vi "Empty.vi"(0 "object in":refnum<class "CetoniPump.lvclass">, 2 "index":i32, 5 "error in (no error)":errorcluster) -> (14 "object out":refnum<class "CetoniPump.lvclass">, 19 "error out":errorcluster)   [LabVIEW 2023, in "CetoniPump.lvclass"]
uses:
  CetoniPump.lvclass
  CetoniPump.lvclass/CetoniPump.ctl
  CETONI_SDK/lib/labview/labbCAN_Pump_API/labbCAN_Pump_API.lvlib
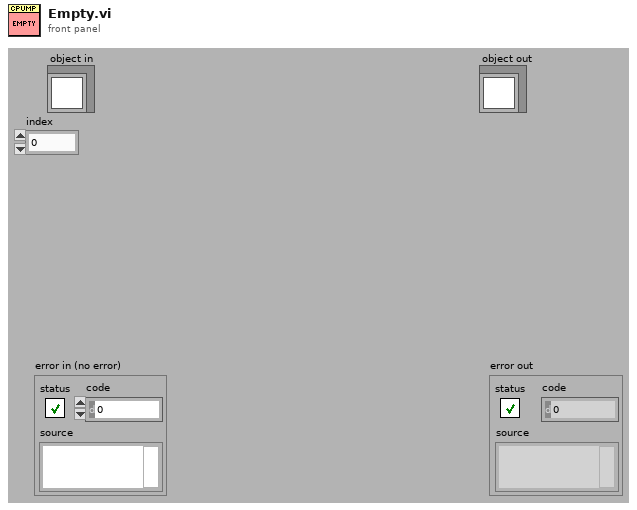
[diagram p1: front panel]
types:
  T1 = cluster{"Pump Handle":i64, "Pump Name":string, "Maximum Volume":dbl, "Maximum Flow Rate":dbl, "Flow Rate":dbl, "Target Level":dbl, "Valve Handle":i64, "Has Valve?":bool, "Actual valve position":i32}[]
  T2 = cluster{"Pump Handle":i64, "Pump Name":string, "Maximum Volume":dbl, "Maximum Flow Rate":dbl, "Flow Rate":dbl, "Target Level":dbl, "Valve Handle":i64, "Has Valve?":bool, "Actual valve position":i32}
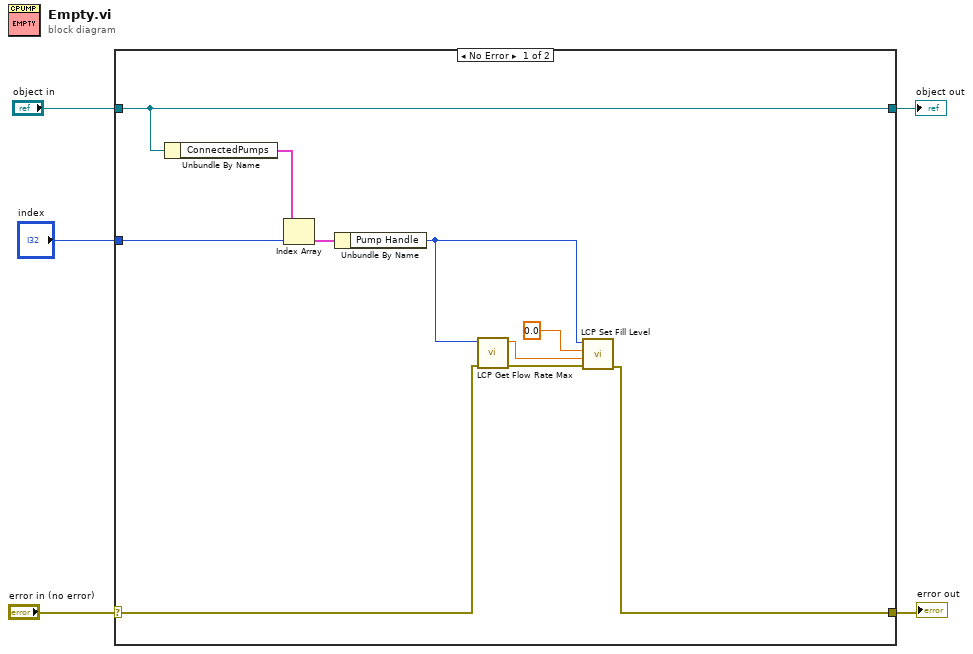
[diagram p0: block diagram]
diagram:
  n1 = case shown="No Error" "error in (no error)" {
    selector: "error in (no error)" -> [w10 w17]
    tunnel: [w9 w17] -> w4
    tunnel: [w15 w16] -> w2
    tunnel: "object in" -> [w15 w16]
    tunnel: "index" -> [w7 _]
    frame No Error {
      n2 = Unbundle By Name(w15) -> ("ConnectedPumps"=w11:T1)
      n3 = Index Array(array=w11, index=w7) -> (element=w8:T2)
      n4 = Unbundle By Name(w8) -> ("Pump Handle"=w6:i64)
      n5 = call "LCP Get Flow Rate Max.vi"("error in (no error)"=w10, "Pump Handle"=w6) -> ("error out"=w14:errorcluster, "Maximum Flow Rate"=w13:dbl)  [unwired: 8 in]
      n6 = call "LCP Set Fill Level.vi"("error in (no error)"=w14, "Flow"=w13, "Level"=0.0, "Pump Handle"=w6) -> ("error out"=w9:errorcluster)  [unwired: 7 in]
    }
    frame Error {
    }
  }
  "error out" <- w4
  "object out" <- w2
